vi "BGK8001 Read.vi"(8 "error in (no error)":errorcluster caption="错误输入（无错误）", 9 "Last Data Array":dbl[](array[numeric])=[0.0, 0.0, 0.0, 0.0, 0.0, 0.0, 0.0, 0.0, 0.0, 0.0, 0.0, 0.0] caption="原数据数组", 11 "VISA Ref Input":refnum<visa-resource-name>="COM2" caption="VISA引用句柄输入") -> (0 "error out":errorcluster caption="错误输出", 1 "New Data Array":dbl[](array[numeric]) caption="新数据数组", 3 "VISA Ref Output":refnum<visa-resource-name> caption="VISA引用句柄输出")   [LabVIEW 2015]
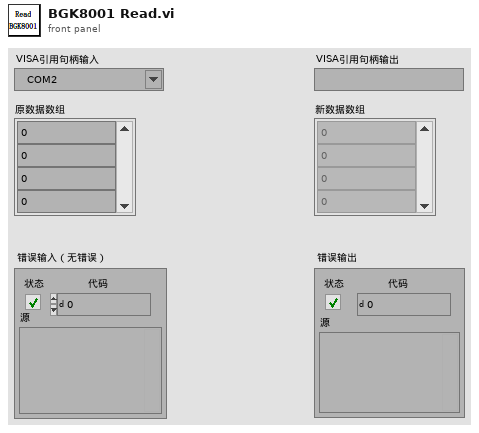
[diagram p1: front panel]
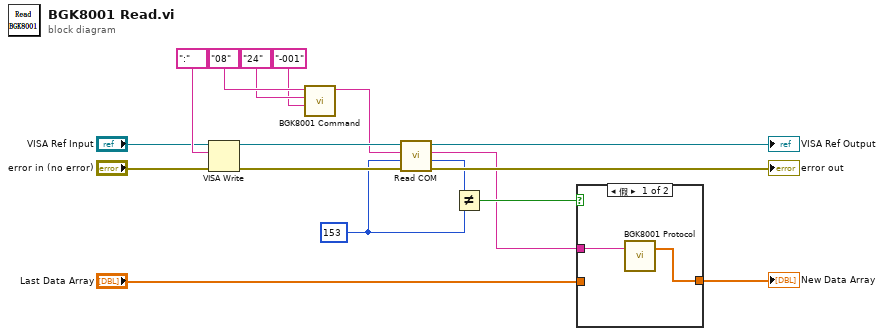
[diagram p0: block diagram]
diagram:
  w6 = u32 153 ("read bytes")
  n1 = VISA Write(VISA resource name="VISA Ref Input", write buffer=":" ("写入缓冲区"), error in (no error)="error in (no error)") -> (VISA resource name out=w14:refnum<visa-resource-name>, error out=w15:errorcluster)  [unwired: 1 out]
  n2 = call "BGK8001 Command.vi"("cmd parameter"="-001" ("格式字符串"), "cmd code"="24", "unit adress"="08") -> ("cmd"=w8:string)  [unwired: 8 in]
  n3 = call "Read COM.vi"("error in"=w15, "read bytes"=w6, "write to buffer"=w8, "VISA resource name in"=w14) -> ("error out"=→"error out":errorcluster, "get bytes"=w1:u32, "read from buffer"=w3:string, "VISA resource name out"=→"VISA Ref Output":refnum<visa-resource-name>)  [unwired: 4 in]
  n4 = Not Equal?(x=w1, y=w6) -> (x != y?=w5:bool)
  n5 = case shown="假" w5 {
    tunnel: [w18 w20] -> w17
    tunnel: w3 -> [w19 _]
    tunnel: "Last Data Array" -> [_ w20]
    frame False {
      n6 = call "BGK8001 Protocol.vi"("字符串"=w19) -> ("数组"=w18:dbl[])  [unwired: 1 in, 1 out]
    }
    frame True {
    }
  }
  "New Data Array" <- w17
